vi "AMZ_S3_AUTH_Add or Replace Date Header.vi"(8 "error in (no error)":errorcluster, 11 "Headers in":T1[](array[typedef])) -> (0 "error out":errorcluster, 3 "Headers":T1[](array[typedef]))   [LabVIEW 2015, in "LV Interface for Amazon S3.lvlib"]
uses:
  LV Interface for Amazon S3.lvlib
  Typedefs/AMZ_S3_HTTP Header-Value pair.ctl
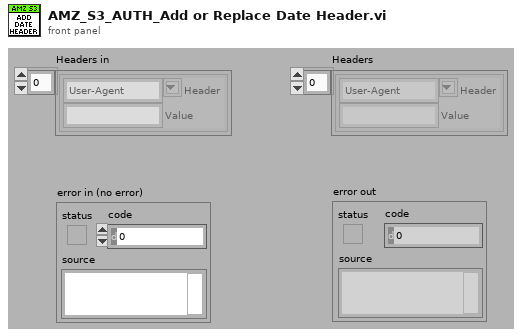
[diagram p1: front panel]
types:
  T1 = typedef "LV Interface for Amazon S3.lvlib/AMZ_S3_HTTP Header-Value pair.ctl" = cluster{"Header":string, "Value":string}
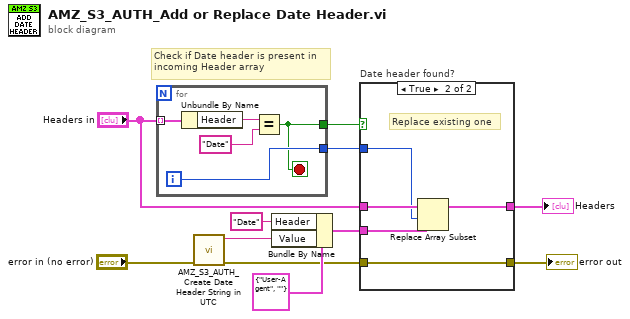
[diagram p0: block diagram]
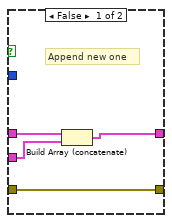
[diagram p2: hidden frame]
diagram:
  # "Check if Date header is present in\nincoming Header array"
  n1 = for {
    tunnel: "Headers in" -> [w16] mode=indexing
    tunnel: [w13] -> w9
    tunnel: [w12] -> w11
    i -> [w13]
    stop <- w12 stop-if-true
    n2 = Unbundle By Name(w16) -> ("Header"=w15:string)
    n3 = Equal?(x=w15, y="Date") -> (x = y?=w12:bool)
  }
  n4 = call "AMZ_S3_AUTH_Create Date Header String in UTC.vi"("error in (no error)"="error in (no error)") -> ("error out"=w4:errorcluster, "DateTime String (UTC)"=w7:string)  [unwired: 9 in]
  n5 = Bundle By Name(cluster=T1 {"Header"="User-Agent", "Value"=""} ("HTTP Header-Value pair"), "Header"="Date", "Value"=w7) -> (w3:T1)
  n6 = case "Date header found?" shown="True" w11 {
    tunnel: "Headers in" -> [w20 w25]
    tunnel: w9 -> [_ w24]
    tunnel: [w18 w23] -> w2
    tunnel: w4 -> [w17 w21]
    tunnel: w3 -> [w19 w22]
    tunnel: [w17 w21] -> w1
    frame False {
      # "Append new one"
      n7 = Build Array (concatenate)(w20, w19) -> (w18:T1[])
    }
    frame True {
      # "Replace existing one"
      n8 = Replace Array Subset(array=w25, new element=w22, index=w24) -> (w23:T1[])
    }
  }
  "Headers" <- w2
  "error out" <- w1
